vi "Begin.vi"() -> (0 "CameraDevRef 2":T1, 1 "CameraDevRef":T1)   [LabVIEW 2011]
doc: "Called before other user functions, this VI is expected to open initial I/O refnums, load in file data, and do all program initialization. Notice that the <B>error out</B> terminal is simply used for data flow. Wiring it to other structures or subVIs ensures that this VI runs first."
uses:
  <vilib>/Rock Robotics/WPI/Camera/WPI_CameraDevRef.ctl
  <vilib>/Rock Robotics/SystemInterfaces/DIO/FPGA_DIOPWMChannel.ctl
  <vilib>/Rock Robotics/WPI/Joystick/WPI_JoystickDeviceEnum.ctl
  <vilib>/Rock Robotics/SystemInterfaces/AI/FPGA_AIChannel.ctl
  <vilib>/Rock Robotics/SystemInterfaces/DIO/FPGA_DIORelayChannel.ctl
  <vilib>/Rock Robotics/SystemInterfaces/DIO/FPGA_DIOChannel.ctl
  <vilib>/Rock Robotics/SystemInterfaces/AI/FPGA_AIGyroChannel.ctl
  <vilib>/Rock Robotics/WPI/Relay/WPI_RelayDirection.ctl
  <vilib>/Rock Robotics/WPI/Encoder/WPI_EncoderType.ctl
  <vilib>/Rock Robotics/WPI/DriverStation/DriverStationLCD/WPI_DriverStationLCDLCDLine.ctl
  <vilib>/Rock Robotics/WPI/MotorControl/WPI_MotorControlOpen Victor.vi
  <vilib>/Rock Robotics/WPI/MotorControl/WPI_MotorControlOpen Jaguar.vi
  Robot Global Data.vi
  <vilib>/Utility/file.llb/Read From Spreadsheet File (DBL).vi
  <vilib>/Rock Robotics/WPI/Counter/WPI_CounterDigitalInputToDigitalSource.vi
  <vilib>/Rock Robotics/SystemInterfaces/Typedef/FPGA_TypedefDigitalModule.ctl
  <vilib>/Rock Robotics/SystemInterfaces/Typedef/FPGA_TypedefAnalogModule.ctl
panel:
  out "Path and file":string
  in  "Balls In Robot At Start":dbl=2.0
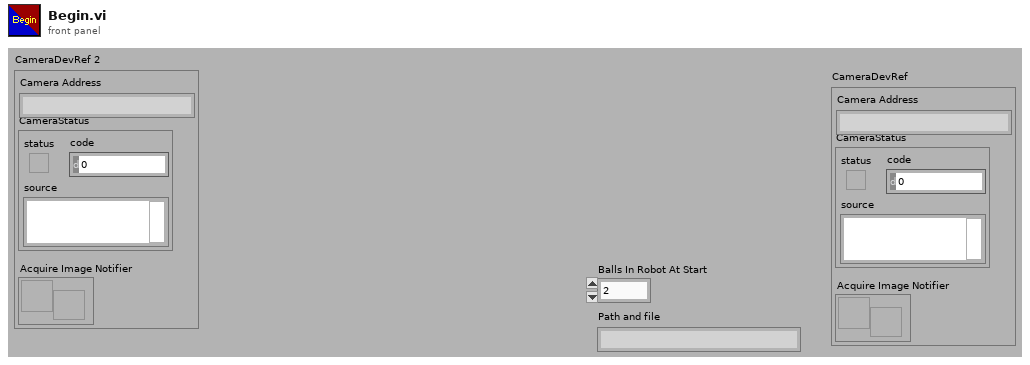
[diagram p1: front panel]
types:
  T1 = typedef "WPI_CameraDevRef.ctl" = cluster{"Camera Address":string, "CameraStatus":errorcluster, "Acquire Image Notifier":refnum<notifier>}
  T2 = typedef "WPI_DriverStationLCDLCDLine.ctl" = enum16{"Main - Line 1", "User - Line 2", "User - Line 3", "User - Line 4", "User - Line 5", "User - Line 6"}
  T3 = typedef "WPI_EncoderType.ctl" = enum16{"1x", "2x", "4x"}
  T4 = typedef "FPGA_DIOChannel.ctl" = enum8{"DIO 1", "DIO 2", "DIO 3", "DIO 4", "DIO 5", "DIO 6", "DIO 7", "DIO 8", "DIO 9", "DIO 10", "DIO 11", "DIO 12", "DIO 13", "DIO 14", "Invalid"}
  T5 = typedef "FPGA_DIORelayChannel.ctl" = enum8{"Relay 1", "Relay 2", "Relay 3", "Relay 4", "Relay 5", "Relay 6", "Relay 7", "Relay 8", "Invalid"}
  T6 = typedef "WPI_RelayDirection.ctl" = enum16{"Both directions", "Forward only", "Reverse only"}
  T7 = typedef "FPGA_AIGyroChannel.ctl" = enum8{"AI 1", "AI 2", "Invalid"}
  T8 = typedef "FPGA_DIOPWMChannel.ctl" = enum8{"PWM 1", "PWM 2", "PWM 3", "PWM 4", "PWM 5", "PWM 6", "PWM 7", "PWM 8", "PWM 9", "PWM 10", "Invalid"}
  T9 = typedef "FPGA_AIChannel.ctl" = enum8{"AI 1", "AI 2", "AI 3", "AI 4", "AI 5", "AI 6", "AI 7", "AI 8", "Invalid"}
  T10 = typedef "WPI_JoystickDeviceEnum.ctl" = enum16{"USB 1", "USB 2", "USB 3", "USB 4", "Kinect 1", "Kinect 2"}
  T11 = typedef "WPI_CameraImageSize.ctl" = enum16{"640x480", "320x240", "160x120"}
  T12 = cluster{"fps":i32, "compression":i32, "Image Size":T11}
  T13 = typedef "WPI_MotorControlDeviceRef.ctl" = cluster{"DeviceStatus":errorcluster, "Type":enum16{"PWM", "CAN"}, "PWM":cluster{"Digital Module":T14, "PWM Channel":T8, "DeadBand":T15}, "CAN":cluster{"Device Number":u8, "Control Mode":T16, "Semaphore":T17, "Max Vout":dbl}, "Invert":bool, "TransformRef":T18, "InvTransformRef":T18}
  T14 = typedef "FPGA_TypedefDigitalModule.ctl" = enum16{"Digital Module 1", "Digital Module 2"}
  T15 = typedef "WPI_PWMDeadband.ctl" = cluster{"Name":string, "maxPositivePwm":i32, "minPositivePwm":i32, "centerPwm":i32, "maxNegativePwm":i32, "minNegativePwm":i32, "angularRange":u16}
  T16 = typedef "WPI_CANJaguar_ControlMode.ctl" = enum8{"Percent VBus", "Current", "Speed", "Position", "Voltage"}
  T17 = typedef "Semaphore RefNum" = refnum<k1>
  T18 = typedef "WPI_PWMTransform_ConPane.ctl" = refnum<vi>
  T19 = typedef "WPI_ServoDeviceRef.ctl" = cluster{"DeviceStatus":errorcluster, "Digital Module":T14, "PWM Channel":T8, "DeadBand":T15}
  T20 = typedef "WPI_AnalogChannelDevRef.ctl" = cluster{"DevStatus":errorcluster, "Analog Module":T21, "Analog Channel":T9}
  T21 = typedef "FPGA_TypedefAnalogModule.ctl" = enum16{"Analog Module 1", "Analog Module 2"}
  T22 = typedef "WPI_CameraWhite Balance Values.ctl" = enum16{"Auto", "Fixed indoor", "Fixed outdoor 1", "Fixed outdoor 2", "Fixed fluorescent 1", "Fixed fluorescent 2", "Hold current"}
  T23 = typedef "WPI_JoystickDevRef.ctl" = cluster{"Device":T10}
  T24 = typedef "WPI_RelayDevRef.ctl" = cluster{"DevStatus":errorcluster, "Relay Channel":T5, "Digital Module":T14, "Relay Direction":T6}
  T25 = typedef "WPI_CameraExposure Values.ctl" = enum16{"Auto", "Flicker-free 50 Hz", "Flicker-free 60 Hz", "Hold current"}
  T26 = typedef "WPI_DigitalInputDevRef.ctl" = cluster{"DevStatus":errorcluster, "DIO Channel":T4, "Digital Module":T14}
  T27 = typedef "FPGA_CounterEncoderSourceConvertionLVSourceType.ctl" = cluster{"DevStatus":errorcluster, "AnalogTriggerMode?":bool, "DigitalMode":cluster{"Digital Module":T14, "DIO Channel":T28}, "AnalogTriggerMode":cluster{"AnalogTriggerIndex":T29, "OutputType":T30}}
  T28 = typedef "FPGA_DIODigitalSourceChannel.ctl" = enum8{"DIO 1", "DIO 2", "DIO 3", "DIO 4", "DIO 5", "DIO 6", "DIO 7", "DIO 8", "DIO 9", "DIO 10", "DIO 11", "DIO 12", "DIO 13", "DIO 14", "Disabled"}
  T29 = typedef "FPGA_AnalogTriggerIndex.ctl" = enum8{"Trig 0", "Trig 1", "Trig 2", "Trig 3", "Trig 4", "Trig 5", "Trig 6", "Trig 7", "Invalid"}
  T30 = typedef "FPGA_AnalogTriggerOutType.ctl" = enum16{"InWindow", "TriggerState", "Rising", "Falling"}
  T31 = typedef "WPI_EncoderDevRef.ctl" = cluster{"DevStatus":errorcluster, "EncoderIndex":T32, "CounterIndex":T33, "DistancePerCount":dbl, "Decoding Type":T3}
  T32 = typedef "FPGA_EncoderIdx.ctl" = enum8{"Enc 0", "Enc 1", "Enc 2", "Enc 3", "Invalid"}
  T33 = typedef "FPGA_CounterCtrSystemIndex.ctl" = enum8{"Ctr 0", "Ctr 1", "Ctr 2", "Ctr 3", "Ctr 4", "Ctr 5", "Ctr 6", "Ctr 7", "Invalid"}
  T34 = typedef "WPI_GyroDevRef.ctl" = cluster{"DevStatus":errorcluster, "Analog Module":T21, "Analog Channel":T9, "Offset":dbl, "Gain (VoltsPerDegree/Second)":dbl}
  T35 = typedef "WPI_UltrasonicDeviceRef.ctl" = cluster{"DevStatus":errorcluster, "Ping Digital Module":T14, "Echo Digital Module":T14, "Ping Channel":T4, "Echo Channel":T4, "CntIndex":T33}
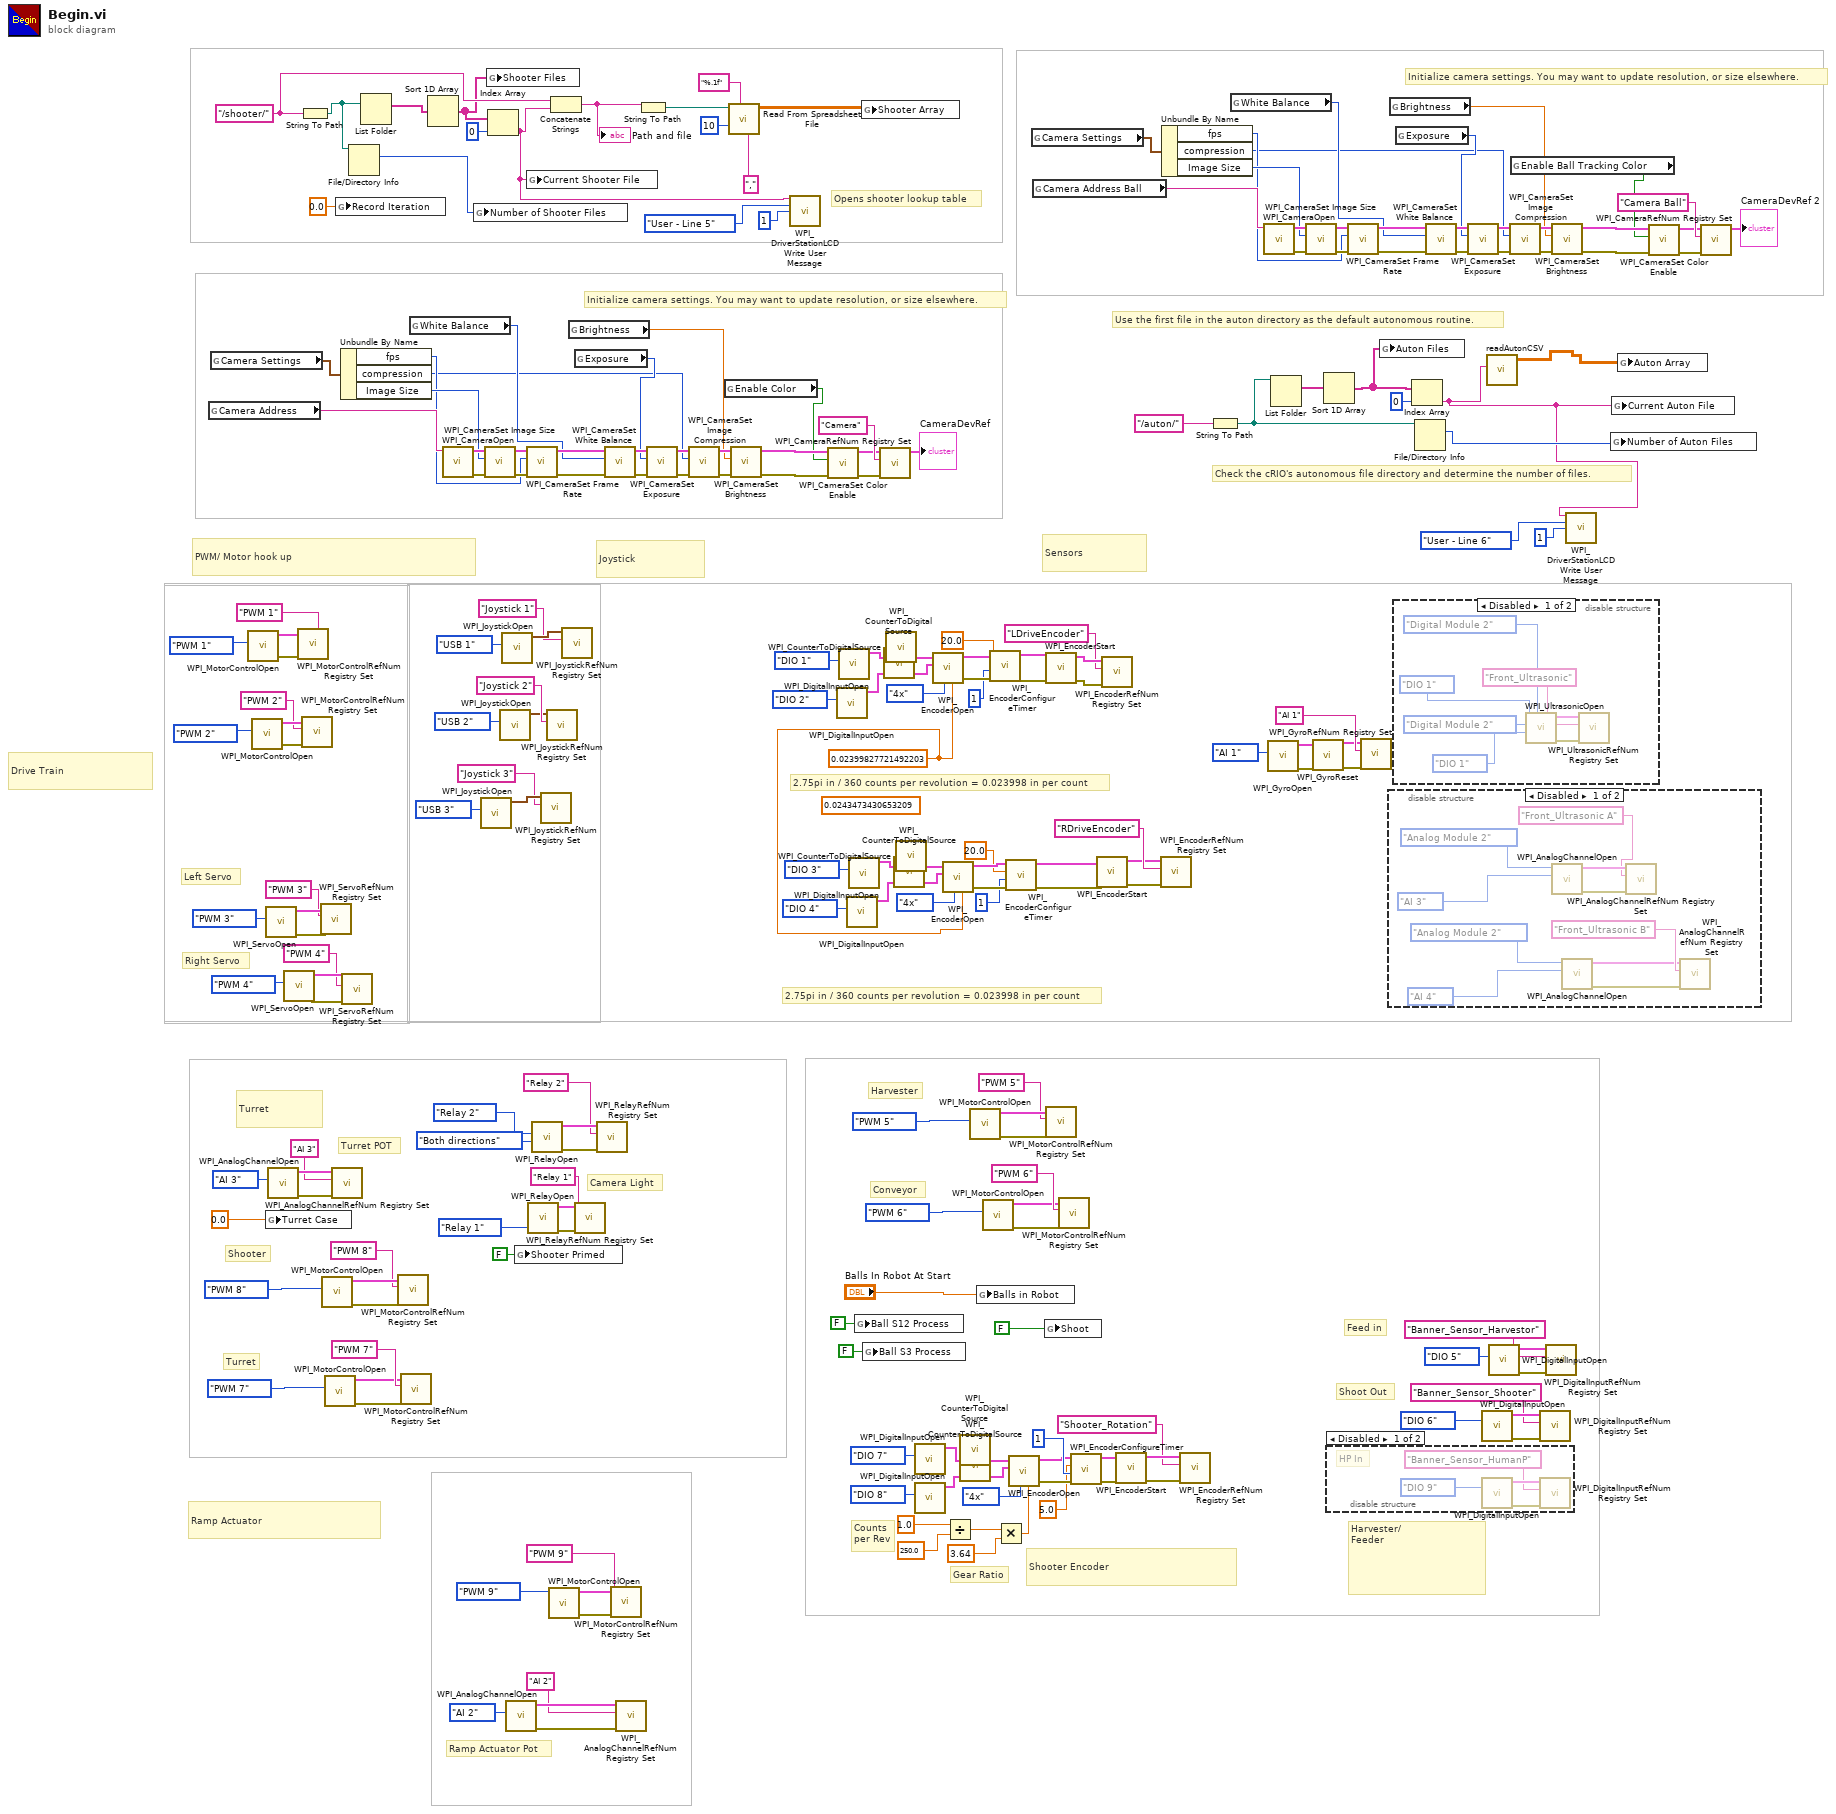
[diagram p0: block diagram]
diagram:
  (unwired) 0.0243473430653209 ("DistancePerCount")
  w58 = 0.02399827721492203 ("DistancePerCount")
  w106 = "/shooter/" ("string")
  # "Shooter Encoder"
  # "Counts\nper Rev"
  # "Gear Ratio"
  # "Initialize camera settings. You may want to update resolution, or size elsewhere."
  # "Check the cRIO's autonomous file directory and determine the number of files."
  # "Use the first file in the auton directory as the default autonomous routine."
  # "2.75pi in / 360 counts per revolution = 0.023998 in per count"
  # "2.75pi in / 360 counts per revolution = 0.023998 in per count"
  # "Opens shooter lookup table"
  # "Shoot Out"
  # "Feed in"
  # "Harvester"
  # "Conveyor"
  # "Shooter"
  # "Initialize camera settings. You may want to update resolution, or size elsewhere."
  # "Camera Light"
  # "Ramp Actuator Pot"
  # "Turret POT"
  # "Turret"
  # "Right Servo"
  # "Left Servo"
  # "Harvester/\nFeeder"
  # "Turret"
  # "Ramp Actuator"
  # "Drive Train"
  # "Sensors"
  # "Joystick"
  # "PWM/ Motor hook up"
  n1 = global read "Robot Global Data.vi" "Camera Address"() -> (w157:string)
  n2 = global read "Robot Global Data.vi" "Camera Settings"() -> (w156:T12)
  n3 = call-poly <vilib>:"WPI_MotorControlOpen.vi"("PWM Channel"=FPGA_DIOPWMChannel."PWM 1") -> ("error out"=w197:errorcluster, "MotorControlDeviceRef"=w199:T13)  [unwired: 9 in]
  n4 = call-poly <vilib>:"WPI_MotorControlOpen.vi"("PWM Channel"=FPGA_DIOPWMChannel."PWM 2") -> ("error out"=w195:errorcluster, "MotorControlDeviceRef"=w193:T13)  [unwired: 9 in]
  n5 = call <vilib>:"WPI_ServoOpen.vi"("PWM Channel"=FPGA_DIOPWMChannel."PWM 3") -> ("error out"=w210:errorcluster, "ServoDeviceRef"=w215:T19)  [unwired: 9 in]
  n6 = global write "Robot Global Data.vi" "Turret Case"(0.0 ("Return To Home Case")) -> ()
  n7 = call <vilib>:"WPI_AnalogChannelOpen.vi"("Analog Channel"=FPGA_AIChannel."AI 3") -> ("error out"=w186:errorcluster, "AIDeviceRef"=w187:T20)  [unwired: 9 in]
  n8 = call <vilib>:"WPI_ServoOpen.vi"("PWM Channel"=FPGA_DIOPWMChannel."PWM 4") -> ("error out"=w209:errorcluster, "ServoDeviceRef"=w213:T19)  [unwired: 9 in]
  n9 = call <vilib>:"WPI_MotorControlRefNum Registry Set.vi"("error in (no error)"=w197, "refnum name"="PWM 1", "MotorControlDevRef"=w199) -> ()  [unwired: 7 in, 2 out]
  n10 = String To Path(string=w106) -> (path=w8:path)
  n11 = call <vilib>:"WPI_MotorControlRefNum Registry Set.vi"("error in (no error)"=w195, "refnum name"="PWM 2", "MotorControlDevRef"=w193) -> ()  [unwired: 7 in, 2 out]
  n12 = call <vilib>:"WPI_ServoRefNum Registry Set.vi"("error in (no error)"=w210, "refnum name"="PWM 3", "ServoDeviceRef"=w215) -> ()  [unwired: 7 in, 2 out]
  n13 = call-poly <vilib>:"WPI_MotorControlOpen.vi"("PWM Channel"=FPGA_DIOPWMChannel."PWM 8") -> ("error out"=w140:errorcluster, "MotorControlDeviceRef"=w142:T13)  [unwired: 9 in]
  n14 = call-poly <vilib>:"WPI_MotorControlOpen.vi"("PWM Channel"=FPGA_DIOPWMChannel."PWM 7") -> ("error out"=w191:errorcluster, "MotorControlDeviceRef"=w189:T13)  [unwired: 9 in]
  n15 = call <vilib>:"WPI_AnalogChannelRefNum Registry Set.vi"("error in (no error)"=w186, "refnum name"="AI 3", "AIDeviceRef"=w187) -> ()  [unwired: 7 in, 2 out]
  n16 = global write "Robot Global Data.vi" "Record Iteration"(0.0 ("Record Iteration")) -> ()
  n17 = Unbundle By Name(w156) -> ("fps"=w154:i32, "compression"=w151:i32, "Image Size"=w155:T11)
  n18 = call <vilib>:"WPI_ServoRefNum Registry Set.vi"("error in (no error)"=w209, "refnum name"="PWM 4", "ServoDeviceRef"=w213) -> ()  [unwired: 7 in, 2 out]
  n19 = File/Directory Info(path=w8) -> (size=w7:i64)  [unwired: 1 in, 6 out]
  n20 = List Folder(path=w8) -> (filenames=w113:string[])  [unwired: 1 in, 5 out]
  n21 = call <vilib>:"WPI_MotorControlRefNum Registry Set.vi"("error in (no error)"=w140, "refnum name"="PWM 8", "MotorControlDevRef"=w142) -> ()  [unwired: 7 in, 2 out]
  n22 = call <vilib>:"WPI_MotorControlRefNum Registry Set.vi"("error in (no error)"=w191, "refnum name"="PWM 7", "MotorControlDevRef"=w189) -> ()  [unwired: 7 in, 2 out]
  n23 = global read "Robot Global Data.vi" "White Balance"() -> (w153:T22)
  n24 = Sort 1D Array(array=w113) -> (sorted array=w9:string[])
  n25 = call <vilib>:"WPI_CameraOpen.vi"("Camera Address"=w157) -> ("error out"=w163:errorcluster, "CameraDevRef"=w164:T1)  [unwired: 1 in, 8 out]
  n26 = global write "Robot Global Data.vi" "Number of Shooter Files"(w7) -> ()
  n27 = call <vilib>:"WPI_JoystickOpen.vi"("JoystickDevice"=WPI_JoystickDeviceEnum."USB 3") -> ("JoystickDevRef"=w202:T23)  [unwired: 10 in]
  n28 = call <vilib>:"WPI_CameraSet Image Size.vi"("error in (no error)"=w163, "Image Size"=w155, "CameraDevRef"=w164) -> ("error out"=w162:errorcluster, "CameraDevRef Out"=w165:T1)  [unwired: 7 out]
  n29 = global write "Robot Global Data.vi" "Shooter Files"(w9) -> ()
  n30 = Index Array(array=w9, index=0) -> (element=w1:string)
  n31 = call <vilib>:"WPI_JoystickOpen.vi"("JoystickDevice"=WPI_JoystickDeviceEnum."USB 2") -> ("JoystickDevRef"=w205:T23)  [unwired: 10 in]
  n32 = call <vilib>:"WPI_JoystickOpen.vi"("JoystickDevice"=WPI_JoystickDeviceEnum."USB 1") -> ("JoystickDevRef"=w208:T23)  [unwired: 10 in]
  n33 = call <vilib>:"WPI_AnalogChannelOpen.vi"("Analog Channel"=FPGA_AIChannel."AI 2") -> ("error out"=w181:errorcluster, "AIDeviceRef"=w182:T20)  [unwired: 9 in]
  n34 = global write "Robot Global Data.vi" "Shooter Primed"(FALSE ("Ball S3 Process")) -> ()
  n35 = global write "Robot Global Data.vi" "Current Shooter File"(w1) -> ()
  n36 = call <vilib>:"WPI_CameraSet Frame Rate.vi"("error in (no error)"=w162, "Frame Rate (fps)"=w154, "CameraDevRef"=w165) -> ("error out"=w161:errorcluster, "CameraDevRef Out"=w167:T1)  [unwired: 7 out]
  n37 = call <vilib>:"WPI_RelayOpen.vi"("Relay Channel"=FPGA_DIORelayChannel."Relay 1") -> ("error out"=w174:errorcluster, "RelayDevRef"=w173:T24)  [unwired: 9 in]
  n38 = call <vilib>:"WPI_RelayOpen.vi"("Relay Direction"=WPI_RelayDirection."Both directions", "Relay Channel"=FPGA_DIORelayChannel."Relay 2") -> ("error out"=w101:errorcluster, "RelayDevRef"=w102:T24)  [unwired: 8 in]
  n39 = call <vilib>:"WPI_JoystickRefNum Registry Set.vi"("refnum name"="Joystick 3", "JoystickDevRef"=w202) -> ()  [unwired: 8 in, 2 out]
  n40 = call <vilib>:"WPI_JoystickRefNum Registry Set.vi"("refnum name"="Joystick 2", "JoystickDevRef"=w205) -> ()  [unwired: 8 in, 2 out]
  n41 = call-poly <vilib>:"WPI_MotorControlOpen.vi"("PWM Channel"=FPGA_DIOPWMChannel."PWM 9") -> ("error out"=w177:errorcluster, "MotorControlDeviceRef"=w178:T13)  [unwired: 9 in]
  n42 = Concatenate Strings(w106, w1) -> (w108:string)
  "Path and file" <- w108
  n43 = call <vilib>:"WPI_JoystickRefNum Registry Set.vi"("refnum name"="Joystick 1", "JoystickDevRef"=w208) -> ()  [unwired: 8 in, 2 out]
  n44 = global read "Robot Global Data.vi" "Brightness"() -> (w150:dbl)
  n45 = global read "Robot Global Data.vi" "Exposure"() -> (w152:T25)
  n46 = call <vilib>:"WPI_RelayRefNum Registry Set.vi"("error in (no error)"=w174, "refnum name"="Relay 1", "RelayDevRef"=w173) -> ()  [unwired: 7 in, 2 out]
  n47 = call <vilib>:"WPI_RelayRefNum Registry Set.vi"("error in (no error)"=w101, "refnum name"="Relay 2", "RelayDevRef"=w102) -> ()  [unwired: 7 in, 2 out]
  n48 = call <vilib>:"WPI_CameraSet White Balance.vi"("error in (no error)"=w161, "White Balance"=w153, "CameraDevRef"=w167) -> ("error out"=w160:errorcluster, "CameraDevRef Out"=w166:T1)  [unwired: 7 out]
  n49 = call <vilib>:"WPI_MotorControlRefNum Registry Set.vi"("error in (no error)"=w177, "refnum name"="PWM 9", "MotorControlDevRef"=w178) -> ()  [unwired: 7 in, 2 out]
  n50 = call <vilib>:"WPI_AnalogChannelRefNum Registry Set.vi"("error in (no error)"=w181, "refnum name"="AI 2", "AIDeviceRef"=w182) -> ()  [unwired: 7 in, 2 out]
  n51 = String To Path(string=w108) -> (path=w107:path)
  n52 = call <vilib>:"WPI_CameraSet Exposure.vi"("error in (no error)"=w160, "Exposure"=w152, "CameraDevRef"=w166) -> ("error out"=w159:errorcluster, "CameraDevRef Out"=w169:T1)  [unwired: 7 out]
  n53 = call <vilib>:"WPI_CameraSet Image Compression.vi"("error in (no error)"=w159, "Compression"=w151, "CameraDevRef"=w169) -> ("error out"=w158:errorcluster, "CameraDevRef Out"=w168:T1)  [unwired: 7 out]
  n54 = global read "Robot Global Data.vi" "Enable Color"() -> (w145:bool)
  n55 = call-poly <vilib>:"Read From Spreadsheet File.vi"("delimiter (\\t)"="," ("delimiter (\\t)"), "format (%.3f)"="%.1f", "number of rows (all:-1)"=10, "file path (dialog if empty)"=w107) -> ("all rows"=w105:dbl[][])  [unwired: 1 in, 6 out]
  n56 = call <vilib>:"WPI_CameraSet Brightness.vi"("error in (no error)"=w158, "Brightness"=w150, "CameraDevRef"=w168) -> ("error out"=w148:errorcluster, "CameraDevRef Out"=w149:T1)  [unwired: 7 out]
  n57 = call <vilib>:"WPI_DriverStationLCDWrite User Message.vi"("line text"=w1, "line"=WPI_DriverStationLCDLCDLine."User - Line 5", "starting column"=i8 1) -> ()  [unwired: 2 in, 11 out]
  n58 = call <vilib>:"WPI_CameraSet Color Enable.vi"("error in (no error)"=w148, "Color Enabled"=w145, "CameraDevRef"=w149) -> ("error out"=w146:errorcluster, "CameraDevRef Out"=w147:T1)  [unwired: 7 in]
  n59 = call <vilib>:"WPI_DigitalInputOpen.vi"("DIO Channel"=FPGA_DIOChannel."DIO 2") -> ("DigitalInputDevRef"=w93:T26)  [unwired: 9 in, 1 out]
  n60 = call <vilib>:"WPI_DigitalInputOpen.vi"("DIO Channel"=FPGA_DIOChannel."DIO 1") -> ("DigitalInputDevRef"=w90:T26)  [unwired: 9 in, 1 out]
  n61 = call <vilib>:"WPI_DigitalInputOpen.vi"("DIO Channel"=FPGA_DIOChannel."DIO 4") -> ("DigitalInputDevRef"=w84:T26)  [unwired: 9 in, 1 out]
  n62 = call <vilib>:"WPI_DigitalInputOpen.vi"("DIO Channel"=FPGA_DIOChannel."DIO 3") -> ("DigitalInputDevRef"=w87:T26)  [unwired: 9 in, 1 out]
  n63 = global write "Robot Global Data.vi" "Ball S12 Process"(FALSE ("Ball S12 Process")) -> ()
  n64 = global write "Robot Global Data.vi" "Shooter Array"(w105) -> ()
  n65 = global write "Robot Global Data.vi" "Ball S3 Process"(FALSE ("Ball S3 Process")) -> ()
  n66 = call <vilib>:"WPI_CameraRefNum Registry Set.vi"("error in (no error)"=w146, "refnum name"="Camera", "CameraDevRef"=w147) -> ("CameraDevRef"=→"CameraDevRef":T1)  [unwired: 8 out]
  n67 = call-poly <vilib>:"WPI_CounterToDigitalSource.vi"("DigitalInputDevRef"=w93) -> ("Digital Source"=w94:T27)  [unwired: 6 in]
  n68 = call-poly <vilib>:"WPI_CounterToDigitalSource.vi"("DigitalInputDevRef"=w90) -> ("Digital Source"=w89:T27)  [unwired: 6 in]
  n69 = call-poly <vilib>:"WPI_CounterToDigitalSource.vi"("DigitalInputDevRef"=w84) -> ("Digital Source"=w83:T27)  [unwired: 6 in]
  n70 = call-poly <vilib>:"WPI_CounterToDigitalSource.vi"("DigitalInputDevRef"=w87) -> ("Digital Source"=w88:T27)  [unwired: 6 in]
  n71 = call <vilib>:"WPI_DigitalInputOpen.vi"("DIO Channel"=FPGA_DIOChannel."DIO 7") -> ("DigitalInputDevRef"=w42:T26)  [unwired: 9 in, 1 out]
  n72 = call <vilib>:"WPI_DigitalInputOpen.vi"("DIO Channel"=FPGA_DIOChannel."DIO 8") -> ("DigitalInputDevRef"=w45:T26)  [unwired: 9 in, 1 out]
  n73 = call <vilib>:"WPI_EncoderOpen.vi"("DistancePerCount"=w58, "Decoding Type"=WPI_EncoderType."4x", "BSource"=w94, "ASource"=w89) -> ("error out"=w62:errorcluster, "EncoderDevRef"=w65:T31)  [unwired: 6 in]
  n74 = call <vilib>:"WPI_EncoderOpen.vi"("DistancePerCount"=w58, "Decoding Type"=WPI_EncoderType."4x", "BSource"=w83, "ASource"=w88) -> ("error out"=w80:errorcluster, "EncoderDevRef"=w79:T31)  [unwired: 6 in]
  n75 = Divide(x=1.0, y=250.0) -> (x/y=w39:dbl)
  n76 = call-poly <vilib>:"WPI_CounterToDigitalSource.vi"("DigitalInputDevRef"=w42) -> ("Digital Source"=w41:T27)  [unwired: 6 in]
  n77 = call-poly <vilib>:"WPI_CounterToDigitalSource.vi"("DigitalInputDevRef"=w45) -> ("Digital Source"=w46:T27)  [unwired: 6 in]
  n78 = call-poly <vilib>:"WPI_MotorControlOpen.vi"("PWM Channel"=FPGA_DIOPWMChannel."PWM 5") -> ("error out"=w136:errorcluster, "MotorControlDeviceRef"=w138:T13)  [unwired: 9 in]
  n79 = global write "Robot Global Data.vi" "Balls in Robot"("Balls In Robot At Start") -> ()
  n80 = call-poly <vilib>:"WPI_MotorControlOpen.vi"("PWM Channel"=FPGA_DIOPWMChannel."PWM 6") -> ("error out"=w135:errorcluster, "MotorControlDeviceRef"=w133:T13)  [unwired: 9 in]
  n81 = call <vilib>:"WPI_EncoderConfigureTimer.vi"("error in (no error)"=w62, "Number Samples to Average"=u8 1, "Minimum Rate"=20.0, "EncoderDevRef"=w65) -> ("error out"=w63:errorcluster, "EncoderDevRef"=w64:T31)  [unwired: 6 in]
  n82 = Multiply(x=w39, y=3.64) -> (x*y=w37:dbl)
  n83 = call <vilib>:"WPI_EncoderConfigureTimer.vi"("error in (no error)"=w80, "Number Samples to Average"=u8 1, "Minimum Rate"=20.0, "EncoderDevRef"=w79) -> ("error out"=w76:errorcluster, "EncoderDevRef"=w77:T31)  [unwired: 6 in]
  n84 = call <vilib>:"WPI_EncoderOpen.vi"("DistancePerCount"=w37, "Decoding Type"=WPI_EncoderType."4x", "BSource"=w46, "ASource"=w41) -> ("error out"=w49:errorcluster, "EncoderDevRef"=w50:T31)  [unwired: 6 in]
  n85 = global read "Robot Global Data.vi" "Camera Settings"() -> (w22:T12)
  n86 = global read "Robot Global Data.vi" "Camera Address Ball"() -> (w23:string)
  n87 = global write "Robot Global Data.vi" "Shoot"(FALSE ("Ball S12 Process")) -> ()
  n88 = call <vilib>:"WPI_EncoderStart.vi"("error in (no error)"=w63, "EncoderDevRef"=w64) -> ("error out"=w97:errorcluster, "EncoderDevRef"=w96:T31)  [unwired: 8 in]
  n89 = call <vilib>:"WPI_MotorControlRefNum Registry Set.vi"("error in (no error)"=w136, "refnum name"="PWM 5", "MotorControlDevRef"=w138) -> ()  [unwired: 7 in, 2 out]
  n90 = call <vilib>:"WPI_MotorControlRefNum Registry Set.vi"("error in (no error)"=w135, "refnum name"="PWM 6", "MotorControlDevRef"=w133) -> ()  [unwired: 7 in, 2 out]
  n91 = call <vilib>:"WPI_EncoderConfigureTimer.vi"("error in (no error)"=w49, "Number Samples to Average"=u8 1, "Minimum Rate"=5.0, "EncoderDevRef"=w50) -> ("error out"=w53:errorcluster, "EncoderDevRef"=w52:T31)  [unwired: 6 in]
  n92 = call <vilib>:"WPI_EncoderStart.vi"("error in (no error)"=w76, "EncoderDevRef"=w77) -> ("error out"=w74:errorcluster, "EncoderDevRef"=w75:T31)  [unwired: 8 in]
  n93 = call <vilib>:"WPI_EncoderRefNum Registry Set.vi"("error in (no error)"=w97, "refnum name"="LDriveEncoder", "EncoderDevRef"=w96) -> ()  [unwired: 7 in, 2 out]
  n94 = call <vilib>:"WPI_EncoderStart.vi"("error in (no error)"=w53, "EncoderDevRef"=w52) -> ("error out"=w55:errorcluster, "EncoderDevRef"=w54:T31)  [unwired: 8 in]
  n95 = call <vilib>:"WPI_EncoderRefNum Registry Set.vi"("error in (no error)"=w74, "refnum name"="RDriveEncoder", "EncoderDevRef"=w75) -> ()  [unwired: 7 in, 2 out]
  n96 = Unbundle By Name(w22) -> ("fps"=w20:i32, "compression"=w17:i32, "Image Size"=w21:T11)
  n97 = call <vilib>:"WPI_EncoderRefNum Registry Set.vi"("error in (no error)"=w55, "refnum name"="Shooter_Rotation", "EncoderDevRef"=w54) -> ()  [unwired: 7 in, 2 out]
  n98 = String To Path(string="/auton/") -> (path=w70:path)
  n99 = global read "Robot Global Data.vi" "White Balance"() -> (w19:T22)
  n100 = call <vilib>:"WPI_CameraOpen.vi"("Camera Address"=w23) -> ("error out"=w29:errorcluster, "CameraDevRef"=w30:T1)  [unwired: 1 in, 8 out]
  n101 = call <vilib>:"WPI_GyroOpen.vi"("Analog Channel"=FPGA_AIGyroChannel."AI 1") -> ("error out"=w116:errorcluster, "GyroDevRef"=w117:T34)  [unwired: 8 in, 1 out]
  n102 = List Folder(path=w70) -> (filenames=w69:string[])  [unwired: 1 in, 5 out]
  n103 = call <vilib>:"WPI_CameraSet Image Size.vi"("error in (no error)"=w29, "Image Size"=w21, "CameraDevRef"=w30) -> ("error out"=w28:errorcluster, "CameraDevRef Out"=w31:T1)  [unwired: 7 out]
  n104 = call <vilib>:"WPI_GyroReset.vi"("error in (no error)"=w116, "GyroDevRef"=w117) -> ("error out"=w115:errorcluster, "GyroDevRef"=w114:T34)  [unwired: 8 in]
  n105 = Sort 1D Array(array=w69) -> (sorted array=w67:string[])
  n106 = disable-structure shown="Disabled" {
    frame Disabled {
      # "HP In"
      n107 = call <vilib>:"WPI_DigitalInputOpen.vi"("DIO Channel"=FPGA_DIOChannel."DIO 9") -> ("error out"=w219:errorcluster, "DigitalInputDevRef"=w218:T26)  [unwired: 9 in]
      n108 = call <vilib>:"WPI_DigitalInputRefNum Registry Set.vi"("error in (no error)"=w219, "refnum name"="Banner_Sensor_HumanP", "DigitalInputDevRef"=w218) -> ()  [unwired: 7 in, 2 out]
    }
    frame Enabled {
    }
  }
  n109 = call <vilib>:"WPI_CameraSet Frame Rate.vi"("error in (no error)"=w28, "Frame Rate (fps)"=w20, "CameraDevRef"=w31) -> ("error out"=w27:errorcluster, "CameraDevRef Out"=w33:T1)  [unwired: 7 out]
  n110 = call <vilib>:"WPI_GyroRefNum Registry Set.vi"("error in (no error)"=w115, "refnum name"="AI 1", "GyroDevRef"=w114) -> ()  [unwired: 7 in, 2 out]
  n111 = global write "Robot Global Data.vi" "Auton Files"(w67) -> ()
  n112 = disable-structure shown="Disabled" {
    frame Disabled {
      n113 = call <vilib>:"WPI_AnalogChannelOpen.vi"("Analog Channel"=FPGA_AIChannel."AI 3", "Analog Module (Module 1)"=FPGA_TypedefAnalogModule."Analog Module 2") -> ("error out"=w226:errorcluster, "AIDeviceRef"=w225:T20)  [unwired: 8 in]
      n114 = call <vilib>:"WPI_AnalogChannelOpen.vi"("Analog Channel"=FPGA_AIChannel."AI 4", "Analog Module (Module 1)"=FPGA_TypedefAnalogModule."Analog Module 2") -> ("error out"=w221:errorcluster, "AIDeviceRef"=w222:T20)  [unwired: 8 in]
      n115 = call <vilib>:"WPI_AnalogChannelRefNum Registry Set.vi"("error in (no error)"=w226, "refnum name"="Front_Ultrasonic A", "AIDeviceRef"=w225) -> ()  [unwired: 7 in, 2 out]
      n116 = call <vilib>:"WPI_AnalogChannelRefNum Registry Set.vi"("error in (no error)"=w221, "refnum name"="Front_Ultrasonic B", "AIDeviceRef"=w222) -> ()  [unwired: 7 in, 2 out]
    }
    frame Enabled {
    }
  }
  n117 = global read "Robot Global Data.vi" "Brightness"() -> (w16:dbl)
  n118 = disable-structure shown="Disabled" {
    frame Disabled {
      n119 = call <vilib>:"WPI_UltrasonicOpen.vi"("Ping Digital Module (Module 1)"=FPGA_TypedefDigitalModule."Digital Module 2", "Echo DIO Channel"=FPGA_DIOChannel."DIO 1", "Echo Digital Module (Module 1)"=FPGA_TypedefDigitalModule."Digital Module 2", "Ping DIO Channel"=FPGA_DIOChannel."DIO 1") -> ("error out"=w237:errorcluster, "UltrasonicDevRef"=w236:T35)  [unwired: 6 in]
      n120 = call <vilib>:"WPI_UltrasonicRefNum Registry Set.vi"("error in (no error)"=w237, "refnum name"="Front_Ultrasonic", "UltrasonicDevRef"=w236) -> ()  [unwired: 7 in, 2 out]
    }
    frame Enabled {
    }
  }
  n121 = global read "Robot Global Data.vi" "Exposure"() -> (w18:T25)
  n122 = Index Array(array=w67, index=0) -> (element=w4:string)
  n123 = File/Directory Info(path=w70) -> (size=w72:i64)  [unwired: 1 in, 6 out]
  n124 = call <vilib>:"WPI_CameraSet White Balance.vi"("error in (no error)"=w27, "White Balance"=w19, "CameraDevRef"=w33) -> ("error out"=w26:errorcluster, "CameraDevRef Out"=w32:T1)  [unwired: 7 out]
  n125 = call <vilib>:"WPI_CameraSet Exposure.vi"("error in (no error)"=w26, "Exposure"=w18, "CameraDevRef"=w32) -> ("error out"=w25:errorcluster, "CameraDevRef Out"=w35:T1)  [unwired: 7 out]
  n126 = call <vilib>:"WPI_DigitalInputOpen.vi"("DIO Channel"=FPGA_DIOChannel."DIO 6") -> ("error out"=w126:errorcluster, "DigitalInputDevRef"=w125:T26)  [unwired: 9 in]
  n127 = call "readAutonCSV.vi"("AutonFile"=w4) -> ("AutonArray"=w66:dbl[][])  [unwired: 7 in]
  n128 = call <vilib>:"WPI_DigitalInputOpen.vi"("DIO Channel"=FPGA_DIOChannel."DIO 5") -> ("error out"=w129:errorcluster, "DigitalInputDevRef"=w128:T26)  [unwired: 9 in]
  n129 = call <vilib>:"WPI_CameraSet Image Compression.vi"("error in (no error)"=w25, "Compression"=w17, "CameraDevRef"=w35) -> ("error out"=w24:errorcluster, "CameraDevRef Out"=w34:T1)  [unwired: 7 out]
  n130 = global read "Robot Global Data.vi" "Enable Ball Tracking Color"() -> (w11:bool)
  n131 = call <vilib>:"WPI_DigitalInputRefNum Registry Set.vi"("error in (no error)"=w126, "refnum name"="Banner_Sensor_Shooter", "DigitalInputDevRef"=w125) -> ()  [unwired: 7 in, 2 out]
  n132 = call <vilib>:"WPI_DigitalInputRefNum Registry Set.vi"("error in (no error)"=w129, "refnum name"="Banner_Sensor_Harvestor", "DigitalInputDevRef"=w128) -> ()  [unwired: 7 in, 2 out]
  n133 = call <vilib>:"WPI_CameraSet Brightness.vi"("error in (no error)"=w24, "Brightness"=w16, "CameraDevRef"=w34) -> ("error out"=w14:errorcluster, "CameraDevRef Out"=w15:T1)  [unwired: 7 out]
  n134 = call <vilib>:"WPI_DriverStationLCDWrite User Message.vi"("line text"=w4, "line"=WPI_DriverStationLCDLCDLine."User - Line 6", "starting column"=i8 1) -> ()  [unwired: 2 in, 11 out]
  n135 = global write "Robot Global Data.vi" "Number of Auton Files"(w72) -> ()
  n136 = global write "Robot Global Data.vi" "Current Auton File"(w4) -> ()
  n137 = global write "Robot Global Data.vi" "Auton Array"(w66) -> ()
  n138 = call <vilib>:"WPI_CameraSet Color Enable.vi"("error in (no error)"=w14, "Color Enabled"=w11, "CameraDevRef"=w15) -> ("error out"=w12:errorcluster, "CameraDevRef Out"=w13:T1)  [unwired: 7 in]
  n139 = call <vilib>:"WPI_CameraRefNum Registry Set.vi"("error in (no error)"=w12, "refnum name"="Camera Ball", "CameraDevRef"=w13) -> ("CameraDevRef"=→"CameraDevRef 2":T1)  [unwired: 8 out]
